vi "Obtain Bucket.vi"(8 "error in (no error)":errorcluster, 10 "Bucket name":string, 11 "AWS Credentials":T1) -> (0 "error out":errorcluster, 3 "Bucket":refnum<class "Bucket.lvclass">)   [LabVIEW 2015, in "NI_AWS_S3.lvlib" / "Bucket.lvclass"]
doc: "Returns the requested bucket. This operation requires the ListAllMyBuckets permission for the account."
uses:
  Bucket.lvclass
  Core/HTTP Request/AWS Credentials.ctl
  Bucket.lvclass/Bucket.ctl
  Read Name.vi
  Core/HTTP Request/HTTP Request.lvclass
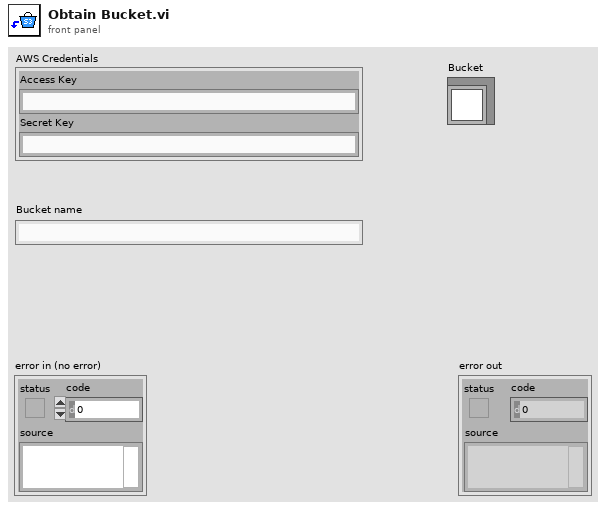
[diagram p1: front panel]
types:
  T1 = typedef "NI_AWS_Core.lvlib/HTTP Request.lvclass/AWS Credentials.ctl" = cluster{"Access Key":string, "Secret Key":string}
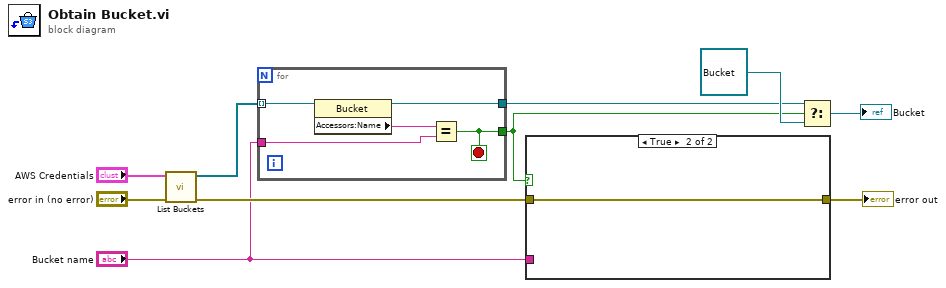
[diagram p0: block diagram]
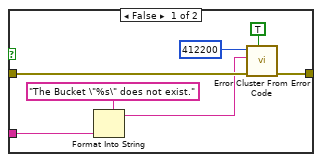
[diagram p2: hidden frame]
diagram:
  n1 = call "List Buckets.vi"("error in (no error)"="error in (no error)", "AWS Credentials"="AWS Credentials") -> ("error out"=w7:errorcluster, "Buckets"=w8:refnum<class "Bucket.lvclass">[])  [unwired: 6 in, 2 out]
  n2 = for {
    tunnel: w8 -> [w15] mode=indexing
    tunnel: "Bucket name" -> [w13]
    tunnel: [w12] -> w3
    tunnel: [w11] -> w4
    stop <- w11 stop-if-true
    n3 = property class="Bucket"(reference=w15) -> (reference out=w12:refnum<class "Bucket.lvclass">, "Accessors:Name"=w14:string)  [unwired: 1 in, 1 out]
    n4 = Equal?(x=w14, y=w13) -> (x = y?=w11:bool)
  }
  n5 = case shown="True" w4 {
    tunnel: w7 -> [w21 w23]
    tunnel: [w22 w23] -> w6
    tunnel: "Bucket name" -> [w17 _]
    frame False {
      n6 = Format Into String(format string="The Bucket \"%s\" does not exist.", w17) -> (resulting string=w16:string)  [unwired: 2 in, 1 out]
      n7 = call <vilib>:"Error Cluster From Error Code.vi"("show call chain? (False)"=TRUE, "error in (no error)"=w21, "error message (\"\")"=w16, "error code (0)"=412200) -> ("error out"=w22:errorcluster)  [unwired: 5 in]
    }
    frame True {
    }
  }
  "error out" <- w6
  n8 = Select(t=w3, s=w4, f=refnum<class "Bucket.lvclass"> refnum ("NI_AWS_S3.lvlib:Bucket.lvclass")) -> (s? t:f=→"Bucket":refnum<class "Bucket.lvclass">)
